vi "Framework Configuration.Contiguous Channel Blocks.vi"(10 "current channel block":T1={"engine offset"=0, "name"="", "data type"=enum."Bool", "count"=1, "buffer offset"=0, "settings"=[]} {"count" format="%d bytes"}, 11 "expected channel block":T1={"engine offset"=0, "name"="", "data type"=enum."Bool", "count"=1, "buffer offset"=0, "settings"=[]} {"count" format="%d bytes"}) -> (3 "contiguous?":bool)   [LabVIEW 2017, in "DSF Core.lvlib" / "Framework Configuration.lvclass"]
uses:
  Framework Configuration.lvclass
  DSF Configuration API/Public/Controls/DSF Engine Channel Configuration.ctl
  DSF Configuration API/Public/Controls/DSF Data Type.ctl
  DSF Configuration API/Public/Controls/DSF Settings Info.ctl
  DSF Core.lvlib
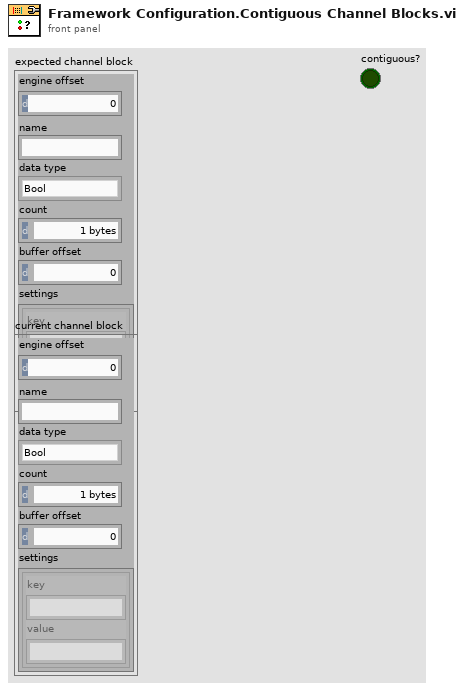
[diagram p1: front panel]
types:
  T1 = typedef "DSF Core.lvlib/DSF Engine Channel Configuration.ctl" = cluster{"engine offset":u64, "name":string, "data type":T2, "count":u64, "buffer offset":u64, "settings":T3}
  T2 = typedef "DSF Core.lvlib/DSF Data Type.ctl" = enum8{"Bool", "SGL", "DBL", "I8", "I16", "I32", "I64", "U8", "U16", "U32", "U64"}
  T3 = typedef "DSF Core.lvlib/DSF Settings Info.ctl" = cluster{"key":string, "value":string}[]
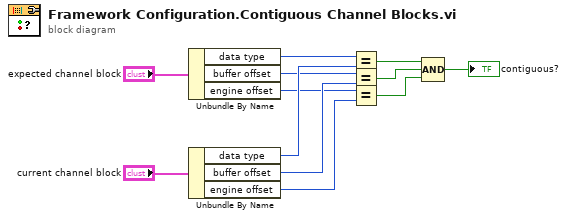
[diagram p0: block diagram]
diagram:
  n1 = Unbundle By Name("expected channel block") -> ("data type"=w10:T2, "buffer offset"=w8:u64, "engine offset"=w6:u64)
  n2 = Unbundle By Name("current channel block") -> ("data type"=w9:T2, "buffer offset"=w7:u64, "engine offset"=w5:u64)
  n3 = Equal?(x=w10, y=w9) -> (x = y?=w4:bool)
  n4 = Equal?(x=w8, y=w7) -> (x = y?=w3:bool)
  n5 = Equal?(x=w6, y=w5) -> (x = y?=w2:bool)
  n6 = Compound Arithmetic op=AND(w4, w3, w2) -> (→"contiguous?":bool)
